vi "sub_do-Multich.vi"(7 "cnt":T1, 8 "error in":errorcluster) -> (0 "error out":errorcluster)   [LabVIEW 2019]
uses:
  cnt_do.ctl
  <vilib>/DAQmx/write.llb/DAQmx Write (Digital 1D Bool NChan 1Samp 1Line).vi
  Durability/common/Global 1.vi
  <vilib>/DAQmx/create/channels.llb/DAQmx Create Channel (DO-Digital Output).vi
  <vilib>/DAQmx/miscellaneous.llb/DAQmx Fill In Error Info.vi
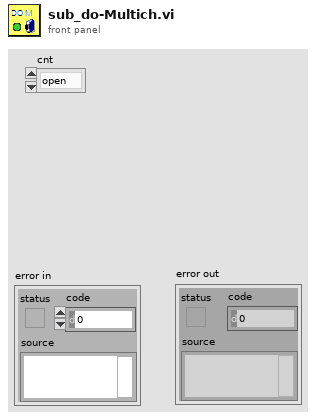
[diagram p1: front panel]
types:
  T1 = typedef "cnt_do.ctl" = enum16{"open", "initial", "update", "run", "close"}
  T2 = typedef "cnt_Relay.ctl" = enum32{"R_Load", "R_out1", "R_out2", "R_out3", "R_out4", "R_out5", "R_out6", "R8", "R9", "R10", "R11", "R12", "R13", "R14", "R15", "R16", "R_in1", "R_in2", "R_in3", "R_in4", "R_in5", "R_in6", "R23", "R24", "R25", "R26", "R27", "R_red", "R_yellow", "R_green", "R_buz", "R_purple"}
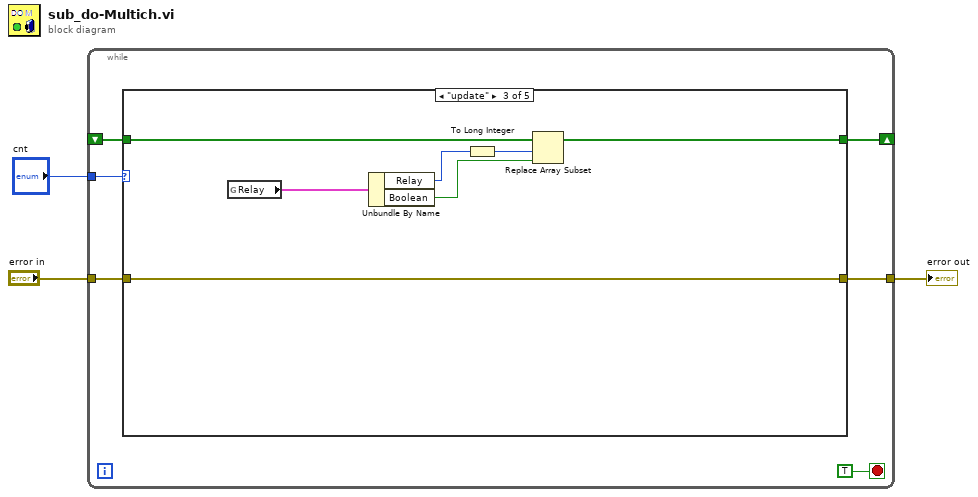
[diagram p0: block diagram]
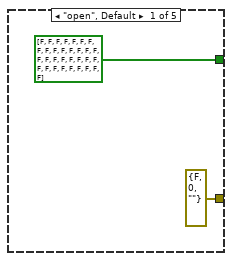
[diagram p2: hidden frame]
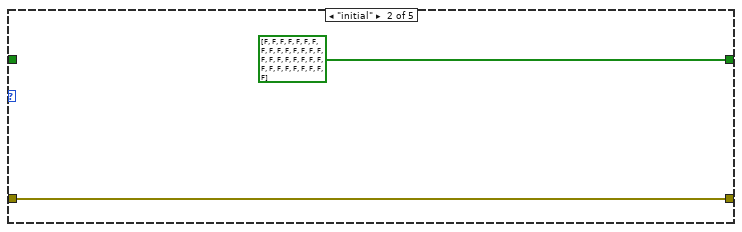
[diagram p3: hidden frame]
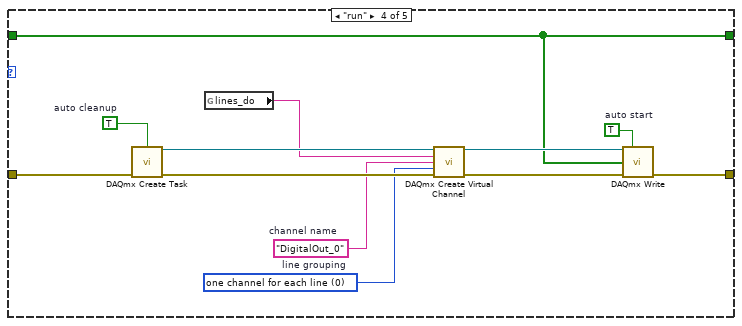
[diagram p4: hidden frame]
diagram:
  n1 = while {
    tunnel: "cnt" -> [w8]
    shift-right: [w7] -> _
    shift-left: _ -> [w6]
    tunnel: "error in" -> [w5]
    tunnel: [w4] -> w1
    stop <- TRUE stop-if-true
    n2 = case shown="\"update\"" w8 {
      tunnel: [bool[] [FALSE, FALSE, FALSE, FALSE, FALSE, FALSE, FALSE, FALSE, FALSE, FALSE, FALSE, FALSE, FALSE, FALSE, FALSE, FALSE, FALSE, FALSE, FALSE, FALSE, FALSE, FALSE, FALSE, FALSE, FALSE, FALSE, FALSE, FALSE, FALSE, FALSE, FALSE, FALSE] ("data") bool[] [FALSE, FALSE, FALSE, FALSE, FALSE, FALSE, FALSE, FALSE, FALSE, FALSE, FALSE, FALSE, FALSE, FALSE, FALSE, FALSE, FALSE, FALSE, FALSE, FALSE, FALSE, FALSE, FALSE, FALSE, FALSE, FALSE, FALSE, FALSE, FALSE, FALSE, FALSE, FALSE] ("data") w19 w24 w34] -> w7
      tunnel: w6 -> [_ _ w20 w24 w34]
      tunnel: w5 -> [_ w12 w18 w23 w33]
      tunnel: [errorcluster {"status"=FALSE, "code"=0, "source"=""} ("error in") w12 w18 w22 w33] -> w4
      frame "open", Default {
      }
      frame "initial" {
      }
      frame "update" {
        n3 = global read "Global 1.vi" "Relay"() -> (w17:cluster{"Relay":T2, "Boolean":bool})
        n4 = Unbundle By Name(w17) -> ("Relay"=w16:T2, "Boolean"=w15:bool)
        n5 = To Long Integer(number=w16) -> (32bit integer=w14:i32)
        n6 = Replace Array Subset(array=w20, new element=w15, index=w14) -> (w19:bool[])
      }
      frame "run" {
        w28 = TRUE  # auto cleanup
        w26 = 0 items=["one channel for each line", "one channel for all lines"]  # line grouping
        w27 = "DigitalOut_0"  # channel name
        w25 = TRUE  # auto start
        n7 = call <vilib>:"DAQmx Create Task.vi"("auto cleanup"=w28, "error in"=w23) -> ("task out"=w30:refnum<k21>, "error out"=w29:errorcluster)  [unwired: 12 in]
        n8 = global read "Global 1.vi" "lines_do"() -> (w21:tag)
        n9 = call-poly <vilib>:"DAQmx Create Virtual Channel.vi"("task in"=w30, "lines"=w21, "name to assign"=w27, "line grouping"=w26, "error in"=w29) -> ("task out"=w31:refnum<k21>, "error out"=w32:errorcluster)  [unwired: 9 in]
        n10 = call-poly <vilib>:"DAQmx Write.vi"("task/channels in"=w31, "auto start"=w25, "data"=w24, "error in"=w32) -> ("error out"=w22:errorcluster)  [unwired: 9 in, 2 out]
      }
      frame "close" {
      }
    }
  }
  "error out" <- w1
